vi "EF_DetectThreshold.vi"(6 "aboveThres_in":bool, 8 "Threshold":u32, 9 "LengthTTrace":u64, 10 "Bin":i32, 11 "TimeTrace":u32[](array[numeric])) -> (3 "aboveThres_out":bool)   [LabVIEW 2017]
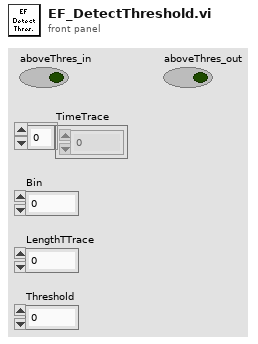
[diagram p1: front panel]
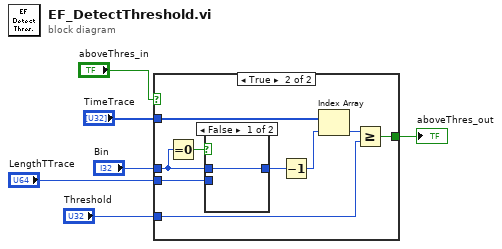
[diagram p0: block diagram]
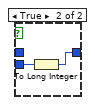
[diagram p3: hidden frame]
diagram:
  n1 = case shown="True" "aboveThres_in" {
    selector: "aboveThres_in" -> [w7 _]
    tunnel: "Threshold" -> [_ w16]
    tunnel: [w7 w15] -> w2
    tunnel: "TimeTrace" -> [_ w13]
    tunnel: "Bin" -> [_ w10]
    tunnel: "LengthTTrace" -> [_ w8]
    frame False {
    }
    frame True {
      n2 = Equal To 0?(x=w10) -> (x = 0?=w12:bool)
      n3 = case shown="False" w12 {
        tunnel: w10 -> [w17 _]
        tunnel: [w17 w18] -> w9
        tunnel: w8 -> [_ w19]
        frame False {
        }
        frame True {
          n4 = To Long Integer(number=w19) -> (32bit integer=w18:i32)
        }
      }
      n5 = Decrement(x=w9) -> (x-1=w11:i32)
      n6 = Index Array(array=w13, index=w11) -> (element=w14:u32)
      n7 = Greater Or Equal?(x=w14, y=w16) -> (x >= y?=w15:bool)
    }
  }
  "aboveThres_out" <- w2
